vi "Untitled 1.vi"() -> ()   [LabVIEW 2013]
panel:
  out "Numeric 2":i32
  out "Numeric":i32
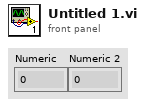
[diagram p1: front panel]
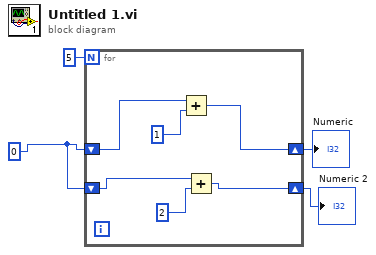
[diagram p0: block diagram]
diagram:
  w2 = 0
  n1 = for {
    N: 5 -> [_]
    shift-right: [w10] -> w3
    shift-left: w2 -> [w9]
    shift-right: [w6] -> w1
    shift-left: w2 -> [w5]
    n2 = Add(x=w9, y=1) -> (x+y=w10:i32)
    n3 = Add(x=w5, y=2) -> (x+y=w6:i32)
  }
  "Numeric" <- w3
  "Numeric 2" <- w1
